vi "Configure Record Parameters (5752).vi"(6 "Record Count":u16=1, 7 "Record Length":u16=3000, 8 "error in":errorcluster, 9 "% of Acquisition Hold Off Time":dbl, 10 "% of Pre-Trigger Samples":dbl, 11 "FPGA VI Reference In":refnum<k20>) -> (0 "error out":errorcluster, 2 "Record Parameters":T1, 3 "FPGA VI Reference Out":refnum<k20>)   [LabVIEW 2012]
uses:
  <vilib>/Utility/error.llb/Error Cluster From Error Code.vi
  <vilib>/rvi/errors/niLvFpgaAdjustHostInterfaceError.vi
  <vilib>/rvi/interface/nirviReadWriteControl/nirviReadWriteControl.xnode
  NiFpgaLv.dll
  <vilib>/rvi/interface/Simulation/niFpgaSimulationCallBeginRW.vi
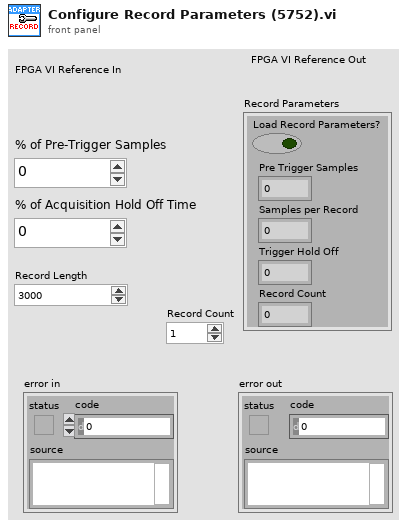
[diagram p1: front panel]
types:
  T1 = cluster{"Load Record Parameters?":bool, "Pre Trigger Samples":u16, "Samples per Record":u16, "Trigger Hold Off":u16, "Record Count":u16}
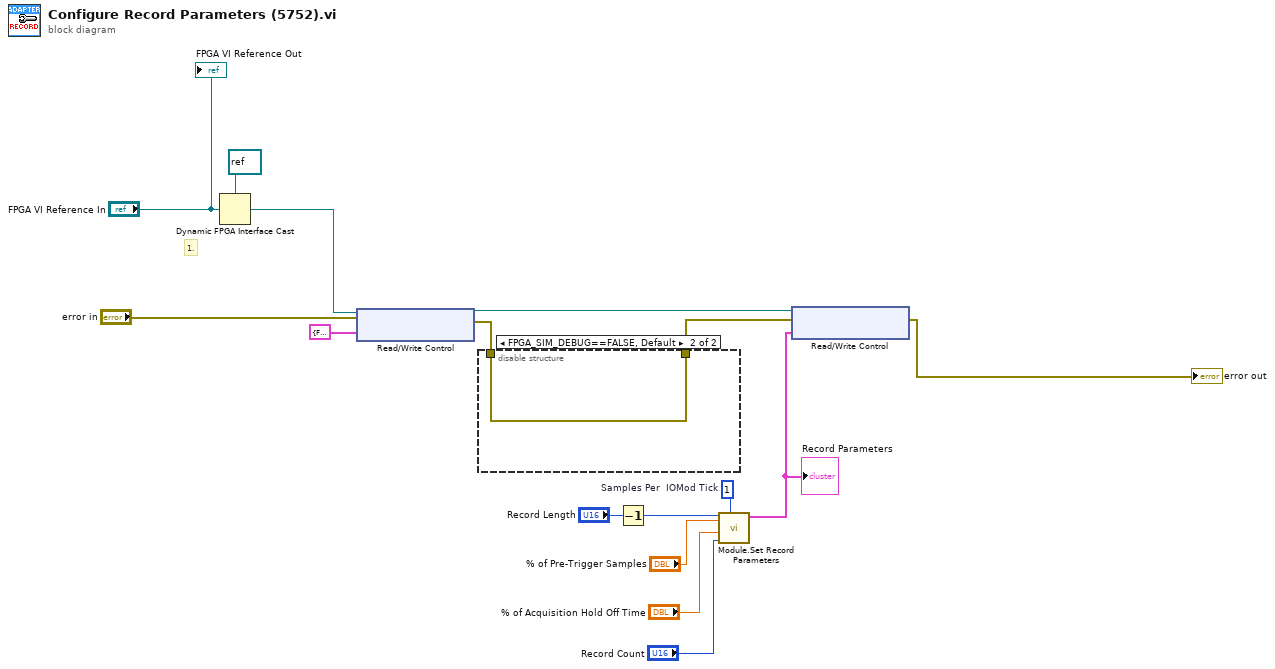
[diagram p0: block diagram]
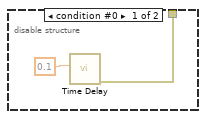
[diagram p2: hidden frame]
diagram:
  w2 = u16 1  # Samples Per  IOMod Tick
  # "1."
  n1 = Dynamic FPGA Interface Cast(Session In=refnum<k20> refnum ("Type"), Type="FPGA VI Reference In") -> (Session Out=w9:refnum<k20>)
  n2 = xnode "Read/Write Control"("FPGA VI Reference In"=w9, "error in"="error in", "Record Parameters"=T1 {"Load Record Parameters?"=FALSE, "Pre Trigger Samples"=0, "Samples per Record"=0, "Trigger Hold Off"=0, "Record Count"=0}) -> ("FPGA VI Reference Out"=w7:refnum<k20>, "error out"=w6:errorcluster)
  n3 = disable-structure shown="FPGA_SIM_DEBUG==FALSE, Default" {
    disable-tunnel: w6 -> [_ w19]
    disable-tunnel: [w17 w19] -> w5
    frame condition #0 {
      n4 = call "Time Delay"("Delay Time (s)"=0.1) -> ("error out"=w17:errorcluster)  [unwired: 10 in]
    }
    frame condition #1 (active) {
    }
  }
  n5 = Decrement(x="Record Length") -> (x-1=w1:u16)
  n6 = call <userlib>:"Module.Set Record Parameters.vi"("Samples Per  IOMod Tick"=w2, "Record Count"="Record Count", "% of Hold Off Time"="% of Acquisition Hold Off Time", "% of Pre-Trigger Samples"="% of Pre-Trigger Samples", "Total Number of Samples"=w1) -> ("Record Parameters"=w4:T1)  [unwired: 3 in, 3 out]
  "Record Parameters" <- w4
  n7 = xnode "Read/Write Control"("FPGA VI Reference In"=w7, "error in"=w5, "Record Parameters"=w4) -> ("error out"=→"error out":errorcluster)  [unwired: 1 out]
  "FPGA VI Reference Out" <- "FPGA VI Reference In"
